vi "Voltage Write.vi"   [LabVIEW 2023, in "Device.lvclass"]
uses:
  Device.lvclass
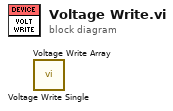
[diagram p0: block diagram]
diagram:
  n1 = call "Voltage Write Single.vi"() -> ()  [unwired: 11 in, 1 out]
  n2 = call "Voltage Write Array.vi"() -> ()  [unwired: 11 in, 1 out]
